vi "SQL_GetAttributesToModify.vi"(8 "error in (no error)":errorcluster, 9 "timeout (15000 ms)":i32=15000, 11 "reference in":refnum<class "SQL.lvclass">) -> (0 "error out":errorcluster, 1 "Timeout":bool, 2 "Attributes":T1, 3 "reference out":refnum<class "SQL.lvclass">)   [LabVIEW 2012, in "SQL.lvclass"]
doc: "This VI returns the attributes associated with this class or subclass object reference and places a lock on the object.\n\nIf the object is currently locked for modification by another method, 'Timeout' specifies how long the VI should wait to receive access to the object. The default value waits until the object becomes available.\n\nYou must use this class SetModifiedAttributes VI to set the object's data and release the lock."
uses:
  SQL.lvclass
  protected/ObjectAttributes.ctl
  <vilib>/addons/database/Connection.llb/Conn ObjectReference.ctl
  Malvern_class/_goop3.llb/3GOOPStates.ctl
  SQL.lvclass/SQL.ctl
  <vilib>/addons/database/NI_Database_API.lvlib
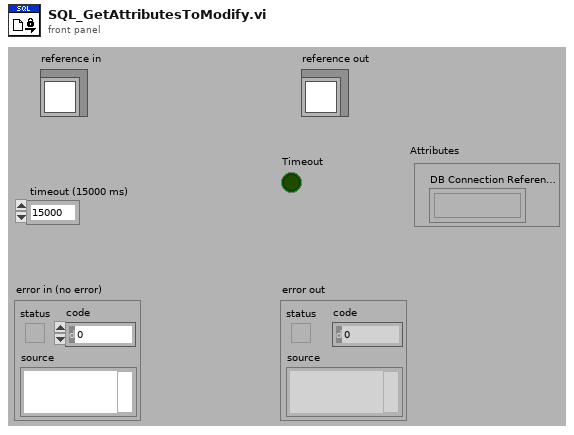
[diagram p1: front panel]
types:
  T1 = typedef "SQL.lvclass/ObjectAttributes.ctl" = cluster{"DB Connection Reference":T2}
  T2 = typedef "NI_Database_API.lvlib/Conn ObjectReference.ctl" = refnum<k1>
  T3 = typedef "3GOOPStates.ctl" = enum16{"Set", "Get", "New", "Delete", "Clear", "Test and get", "Unlock data", "Information", "Look up existing", "New or look up existing", "Test and get shared", "Get shared", "Set shared", "Unlock shared", "Find dynamic method", "Register dynamic method", "Preload dynamic method", "Probe", "Cast to more generic", "Cast to more specific"}
  T4 = typedef "SQL.lvclass/ObjectReference.ctl" = refnum<k1>
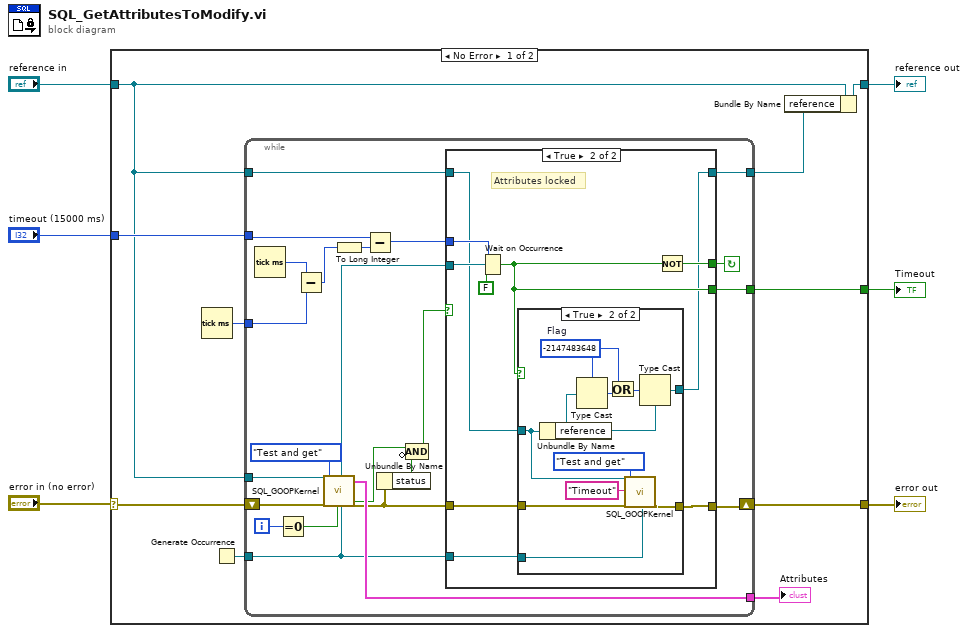
[diagram p0: block diagram]
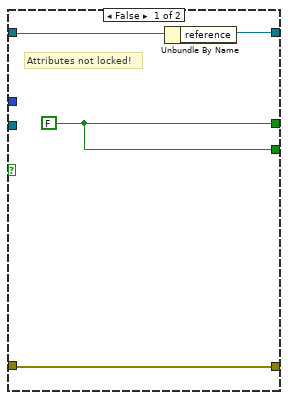
[diagram p2: hidden frame]
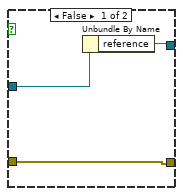
[diagram p3: hidden frame]
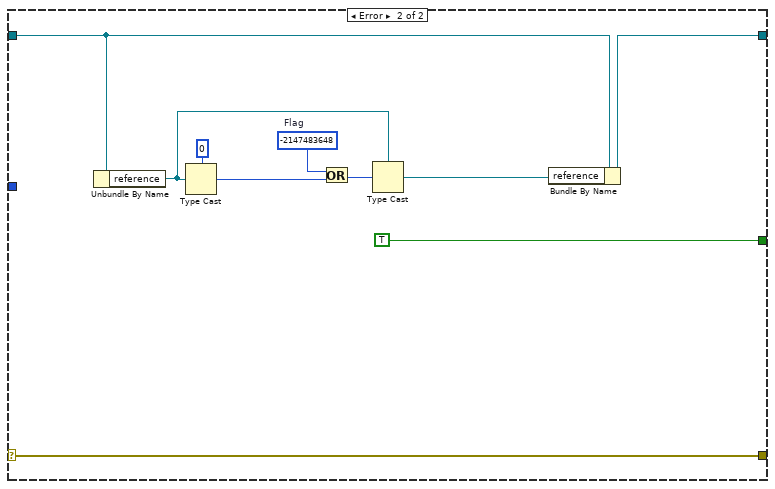
[diagram p4: hidden frame]
diagram:
  n1 = case shown="No Error" "error in (no error)" {
    selector: "error in (no error)" -> [w13 w77]
    tunnel: [w10 w73] -> w6
    tunnel: [w12 w77] -> w5
    tunnel: "reference in" -> [w8 w74]
    tunnel: [w11 TRUE ("timed out")] -> w2
    tunnel: "timeout (15000 ms)" -> [w14 _]
    frame No Error {
      n2 = Tick Count (ms)() -> (millisecond timer value=w15:u32)
      n3 = Generate Occurrence() -> (w16:refnum<k4>)
      n4 = while {
        tunnel: [w35] -> w9
        shift-left: w13 -> [w36]
        shift-right: [w21] -> w12
        tunnel: [w38] -> w11
        tunnel: w14 -> [w27]
        tunnel: w8 -> [w37]
        tunnel: w16 -> [w20]
        tunnel: w15 -> [w17]
        tunnel: w8 -> [w23]
        tunnel: [w19] -> w7
        i -> [w31]
        stop <- w39 continue-if-true
        n5 = Tick Count (ms)() -> (millisecond timer value=w18:u32)
        n6 = Equal To 0?(x=w31) -> (x = 0?=w30:bool)
        n7 = Subtract(x=w18, y=w17) -> (x-y=w26:u32)
        n8 = call "SQL_GOOPKernel.vi"("Ref in"=w37, "error in (no error)"=w36, "Action"=3GOOPStates."Test and get", "Misc"=w30, "Occurrence"=w20) -> ("Occurrence out"=w29:refnum<k4>, "Data out"=w35:T1, "Data locked?"=w33:bool, "error out"=w22:errorcluster)  [unwired: 12 in, 7 out]
        n9 = To Long Integer(number=w26) -> (32bit integer=w24:i32)
        n10 = Subtract(x=w27, y=w24) -> (x-y=w25:i32)
        n11 = Unbundle By Name(w22) -> ("status"=w34:bool)
        n12 = Compound Arithmetic op=AND(w33, invert w34) -> (w32:bool)
        n13 = case shown="True" w32 {
          tunnel: w29 -> [_ w52]
          tunnel: w25 -> [_ w50]
          tunnel: [w43 w53] -> w39
          tunnel: [w43 w46] -> w38
          tunnel: w23 -> [w41 w49]
          tunnel: w22 -> [w42 w48]
          tunnel: [w42 w47] -> w21
          tunnel: w20 -> [_ w45]
          tunnel: [w40 w44] -> w19
          frame False {
            w43 = FALSE
            # "Attributes not locked!"
            n14 = Unbundle By Name(w41) -> ("reference"=w40:T4)
          }
          frame True {
            # "Attributes locked"
            n15 = Wait on Occurrence(1:FALSE ("ignore previous (T)"), 2:w52, 3:w50) -> (0:w46:bool)
            n16 = case shown="True" w46 {
              tunnel: w49 -> [w55 w61]
              tunnel: w48 -> [w56 w67]
              tunnel: [w56 w66] -> w47
              tunnel: w45 -> [_ w64]
              tunnel: [w54 w59] -> w44
              frame False {
                n17 = Unbundle By Name(w55) -> ("reference"=w54:T4)
              }
              frame True {
                w57 = -2147483648  # Flag
                n18 = Unbundle By Name(w61) -> ("reference"=w60:T4)
                n19 = Type Cast(type=w57, x=w60) -> (*(type *) &x=w62:i32)
                n20 = Or(x=w57, y=w62) -> (x .or. y?=w58:i32)
                n21 = call "SQL_GOOPKernel.vi"("Ref in"=w61, "Probe in"="Timeout" ("VI ref"), "error in (no error)"=w67, "Action"=3GOOPStates."Test and get", "Occurrence"=w64) -> ("error out"=w66:errorcluster)  [unwired: 12 in, 10 out]
                n22 = Type Cast(type=w60, x=w58) -> (*(type *) &x=w59:T4)
              }
            }
            n23 = Not(x=w46) -> (.not. x?=w53:bool)
          }
        }
      }
      "Attributes" <- w9
      n24 = Bundle By Name(cluster=w8, "reference"=w7) -> (w10:refnum<class "SQL.lvclass">)
    }
    frame Error {
      w75 = -2147483648  # Flag
      n25 = Unbundle By Name(w74) -> ("reference"=w68:T4)
      n26 = Type Cast(type=0, x=w68) -> (*(type *) &x=w71:i32)
      n27 = Or(x=w75, y=w71) -> (x .or. y?=w70:i32)
      n28 = Type Cast(type=w68, x=w70) -> (*(type *) &x=w69:T4)
      n29 = Bundle By Name(cluster=w74, "reference"=w69) -> (w73:refnum<class "SQL.lvclass">)
    }
  }
  "error out" <- w5
  "reference out" <- w6
  "Timeout" <- w2
